vi "View File.vi"() -> ()   [LabVIEW 2015]
panel:
  out "XY Graph 2":cluster{dbl[], dbl[]}[](graph)
  out "XY Graph":cluster{dbl[], dbl[]}(graph)
  in  "File Path Control":path=path "E:/Data/GloveBox/Boris/tablestage/1_test/June_2016/061416/300.38000K_290_700_0.20000V_0.00000T_Jun14-2016__16-32-28_001_061416.bin"
  out "Waveform Graph":dbl[](graph)
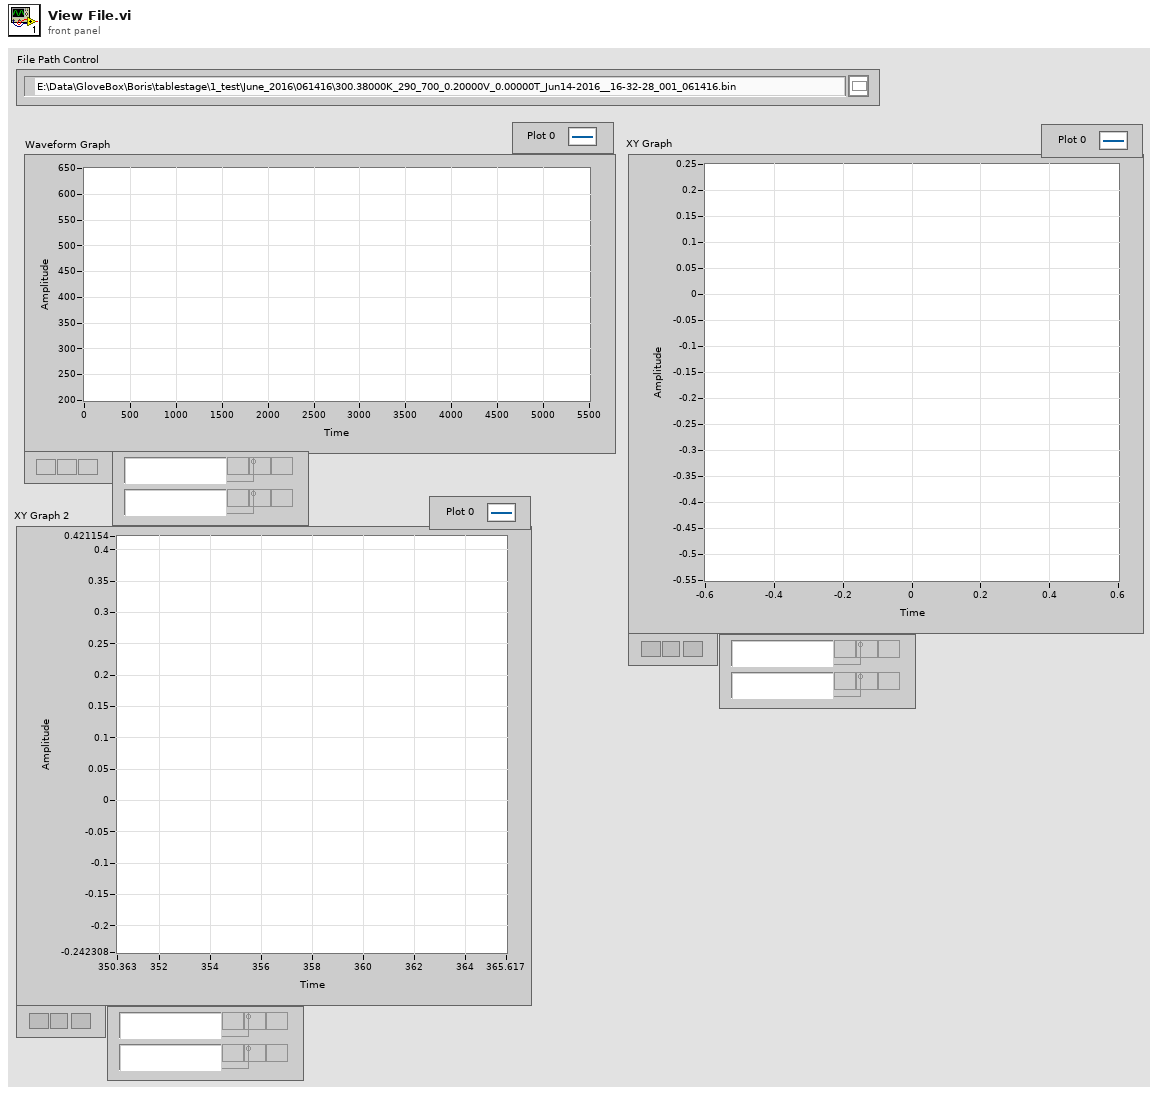
[diagram p1: front panel]
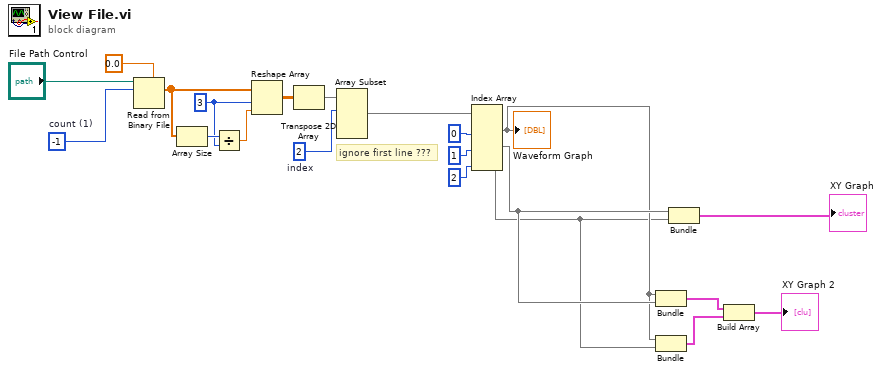
[diagram p0: block diagram]
diagram:
  w8 = 3 ("y")
  w12 = 2  # index
  w21 = -1  # count (1)
  # "ignore first line ???"
  n1 = Read from Binary File(5:0.0, 10:w21, 11:"File Path Control") -> (2:w18:dbl[])  [unwired: 3 in, 3 out]
  n2 = Array Size(array=w18) -> (size(s)=w17:i32)
  n3 = Divide(x=w17, y=w8) -> (x/y=w16:dbl)
  n4 = Reshape Array(w18, w8, w16) -> (w19:dbl[][])
  n5 = Transpose 2D Array(2D array=w19) -> (transposed array=w11:dbl[][])
  n6 = Array Subset(array=w11, index (row)=w12) -> (w10:dbl[][])  [unwired: 3 in]
  n7 = Index Array(array=w10, index (col) #1=0 ("disabled index (col)"), index (col) #2=1 ("disabled index (col)"), index (col) #3=2 ("disabled index (col)")) -> (element #1=w5:dbl[], element #2=w6:dbl[], element #3=w4:dbl[])  [unwired: 3 in]
  "Waveform Graph" <- w5
  n8 = Bundle(w5, w6) -> (w3:cluster{dbl[], dbl[]})  [unwired: 1 in]
  n9 = Bundle(w5, w4) -> (w2:cluster{dbl[], dbl[]})  [unwired: 1 in]
  n10 = Bundle(w6, w4) -> (→"XY Graph":cluster{dbl[], dbl[]})  [unwired: 1 in]
  n11 = Build Array(w3, w2) -> (→"XY Graph 2":cluster{dbl[], dbl[]}[])
